vi "HandlePause.vi"(8 "error in (no error)":errorcluster, 11 "Acquisition in":refnum<class "Acquisition.lvclass">) -> (0 "error out":errorcluster, 2 "pause?":bool, 3 "Acquisition out":refnum<class "Acquisition.lvclass">)   [LabVIEW 2018, in "Acquisition.lvclass"]
uses:
  Acquisition.lvclass
  C:/Users/devstaff/sparc4/s4gui/Versao ZeroMQ REQ-REP/SPARC4_GUI -v1.0.0/Server/Server.lvclass
  Server/Server.lvclass/Server.ctl
  Acquisition.lvclass/Acquisition.ctl
  Channel/Channel.lvclass
  StateMachine/State Machine.lvclass
  Server/Server.lvclass
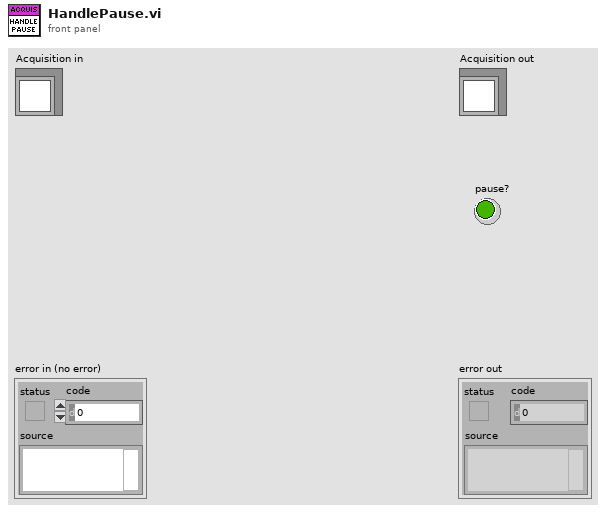
[diagram p1: front panel]
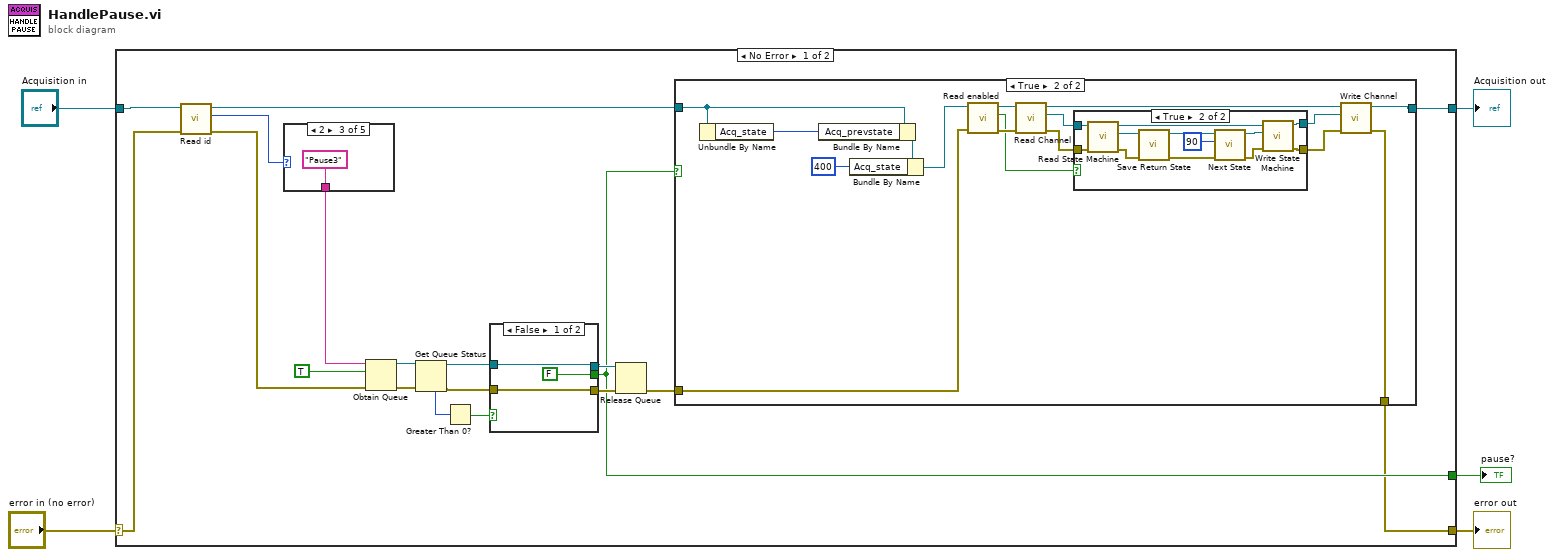
[diagram p0: block diagram]
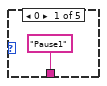
[diagram p2: hidden frame]
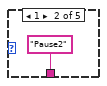
[diagram p3: hidden frame]
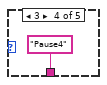
[diagram p4: hidden frame]
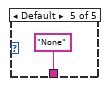
[diagram p5: hidden frame]
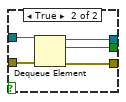
[diagram p8: hidden frame]
diagram:
  n1 = case shown="No Error" "error in (no error)" {
    selector: "error in (no error)" -> [w7 w71]
    tunnel: [w8 w71] -> w4
    tunnel: [w24 w70] -> w2
    tunnel: "Acquisition in" -> [w23 w70]
    tunnel: [w11 _] -> w1
    frame No Error {
      n2 = call "Read id.vi"("error in (no error)"=w7, "Server in"=w23) -> ("error out"=w6:errorcluster, "id"=w10:u32, "Server out"=w22:refnum<class "Acquisition.lvclass">)  [unwired: 7 in]
      n3 = case shown="2" w10 {
        tunnel: ["Pause1" ("name (unnamed)") "Pause2" ("name (unnamed)") "Pause3" ("name (unnamed)") "Pause4" ("name (unnamed)") "None" ("name (unnamed)")] -> w21
        frame 0 {
        }
        frame 1 {
        }
        frame 2 {
        }
        frame 3 {
        }
        frame Default {
        }
      }
      n4 = Obtain Queue(name (unnamed)=w21, element data type=TRUE, error in (no error)=w6) -> (queue out=w18:refnum<queue>, error out=w19:errorcluster)  [unwired: 2 in, 1 out]
      n5 = Get Queue Status(queue=w18, error in (no error)=w19) -> (queue out=w15:refnum<queue>, error out=w14:errorcluster, # elements in queue=w17:i32)  [unwired: 1 in, 5 out]
      n6 = Greater Than 0?(x=w17) -> (x > 0?=w16:bool)
      n7 = case shown="False" w16 {
        tunnel: w15 -> [w63 w68]
        tunnel: w14 -> [w62 w69]
        tunnel: [FALSE w67] -> w11
        tunnel: [w63 w66] -> w13
        tunnel: [w62 w65] -> w12
        frame False {
        }
        frame True {
          n8 = Dequeue Element(queue=w68, error in (no error)=w69) -> (queue out=w66:refnum<queue>, element=w67:bool, error out=w65:errorcluster)  [unwired: 1 in, 1 out]
        }
      }
      n9 = Release Queue(queue=w13, error in (no error)=w12) -> (error out=w9:errorcluster)  [unwired: 1 in, 2 out]
      n10 = case shown="True" w11 {
        tunnel: [w31 w42] -> w24
        tunnel: w22 -> [w31 w47]
        tunnel: w9 -> [w30 w34]
        tunnel: [w30 w39] -> w8
        frame False {
        }
        frame True {
          n11 = Unbundle By Name(w47) -> ("Acq_state"=w46:u32)
          n12 = Bundle By Name(cluster=w47, "Acq_prevstate"=w46) -> (w45:refnum<class "Acquisition.lvclass">)
          n13 = Bundle By Name(cluster=w45, "Acq_state"=u32 400) -> (w35:refnum<class "Acquisition.lvclass">)
          n14 = call-dynamic "Read enabled.vi"("error in (no error)"=w34, "Server in"=w35) -> ("error out"=w33:errorcluster, "enabled"=w32:bool, "Server out"=w36:refnum<class "Acquisition.lvclass">)  [unwired: 7 in]
          n15 = call-dynamic "Read Channel.vi"("error in (no error)"=w33, "Acquisition in"=w36) -> ("error out"=w37:errorcluster, "Channel.lvclass"=w38:refnum<class "Channel.lvclass">, "Acquisition out"=w41:refnum<class "Acquisition.lvclass">)  [unwired: 7 in]
          n16 = case shown="True" w32 {
            tunnel: w38 -> [w49 w61]
            tunnel: [w49 w59] -> w40
            tunnel: w37 -> [w48 w54]
            tunnel: [w48 w50] -> w43
            frame False {
            }
            frame True {
              n17 = call-dynamic "Read State Machine.vi"("error in (no error)"=w54, "Device in"=w61) -> ("error out"=w53:errorcluster, "State Machine.lvclass"=w58:refnum<class "State Machine.lvclass">, "Device out"=w60:refnum<class "Channel.lvclass">)  [unwired: 7 in]
              n18 = call-dynamic "Save Return State.vi"("error in (no error)"=w53, "State Machine in"=w58) -> ("error out"=w52:errorcluster, "State Machine out"=w57:refnum<class "State Machine.lvclass">)  [unwired: 8 in]
              n19 = call "Next State.vi"("error in (no error)"=w52, "New_State"=90, "State Machine in"=w57) -> ("error out"=w51:errorcluster, "State Machine out"=w56:refnum<class "State Machine.lvclass">)  [unwired: 7 in]
              n20 = call-dynamic "Write State Machine.vi"("error in (no error)"=w51, "State Machine.lvclass"=w56, "Device in"=w60) -> ("error out"=w50:errorcluster, "Device out"=w59:refnum<class "Channel.lvclass">)  [unwired: 7 in]
            }
          }
          n21 = call-dynamic "Write Channel.vi"("error in (no error)"=w43, "Channel.lvclass"=w40, "Acquisition in"=w41) -> ("error out"=w39:errorcluster, "Acquisition out"=w42:refnum<class "Acquisition.lvclass">)  [unwired: 7 in]
        }
      }
    }
    frame Error {
    }
  }
  "error out" <- w4
  "Acquisition out" <- w2
  "pause?" <- w1
